vi "Get ctrl Secondary Button.vi"(3 "Button Secondary":T1(ring)) -> (0 "Button Secondary":bool)   [LabVIEW 2014]
uses:
  SRE Enum.ctl
  Support Code/Robot Global Data.vi
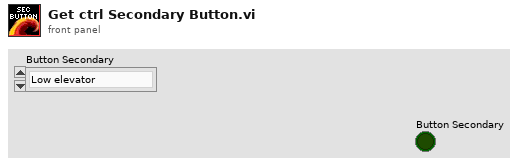
[diagram p1: front panel]
types:
  T1 = enum16{"Low elevator", "High elevator", "Claw up", "Claw Down", "Open/Close claw"}
  T2 = typedef "SRE Enum.ctl" = enum16{"Start", "Run", "End"}
  T3 = enum16{"Left X", "Left Y", "Left trigger", "R trigger", "R X", "R Y"}[]
  T4 = enum16{"Left X", "Left Y", "Left trigger", "R trigger", "R X", "R Y"}
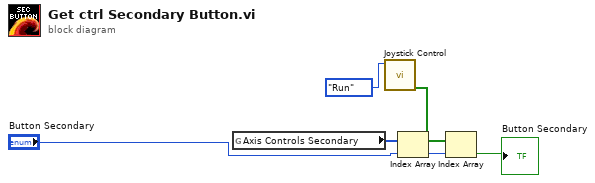
[diagram p0: block diagram]
diagram:
  n1 = global read "Robot Global Data.vi" "Axis Controls Secondary"() -> (w6:T3)
  n2 = call "Joystick Control.vi"("Enum"=SRE_Enum."Run") -> ("Buttons Output Secondary"=w2:bool[])  [unwired: 3 in, 5 out]
  n3 = Index Array(array=w6, index="Button Secondary") -> (element=w5:T4)
  n4 = Index Array(array=w2, index=w5) -> (element=→"Button Secondary":bool)
